vi "Uninitialize.vi"(8 "error in":errorcluster) -> (0 "error out":errorcluster)   [LabVIEW 2019]
doc: "Removes all VIs from registry, deletes the current language and the dictionary."
uses:
  SubVIs/Localization FGV Action -- Enum.ctl
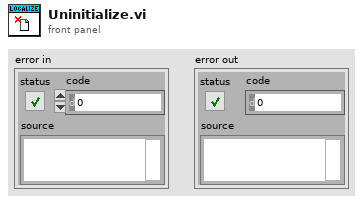
[diagram p1: front panel]
types:
  T1 = typedef "Localization FGV Action -- Enum.ctl" = enum16{"Read Dictionary", "Translate VIs", "Register VI", "Get Languages", "Translate Phrase", "Get Key For Phrase", "Get Phrase For Phrase", "Translate VI", "Unregister"}
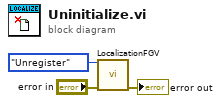
[diagram p0: block diagram]
diagram:
  n1 = call "LocalizationFGV.vi"("Action"=Localization_FGV_Action_--_Enum."Unregister", "error in"="error in") -> ("error out"=→"error out":errorcluster)  [unwired: 8 in, 5 out]
